vi "compressor.vi"() -> ()   [LabVIEW 2017]
uses:
  <vilib>/Rock Robotics/WPI/Utilities/WPI_GetSetVariantRefNum.vi
panel:
  out "Compressor Enabled":bool
  out "Compressor Running":bool
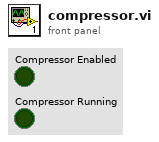
[diagram p1: front panel]
types:
  T1 = typedef "WPI_CompressorDevRef.ctl" = cluster{"DevStatus":errorcluster, "Pneumatics Control Module":u8}
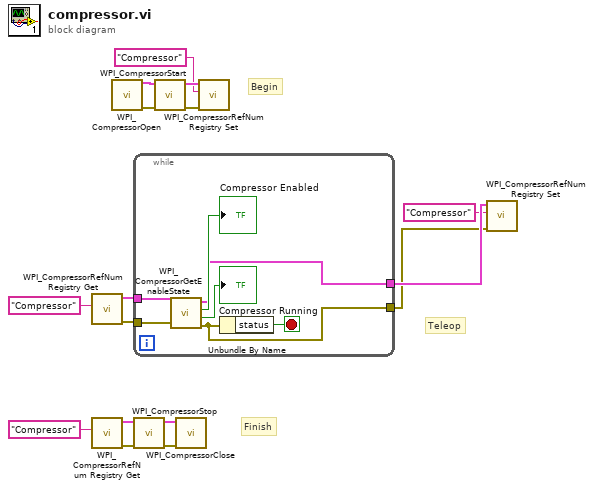
[diagram p0: block diagram]
diagram:
  # "Begin"
  # "Finish"
  # "Teleop"
  n1 = call <vilib>:"WPI_CompressorRefNum Registry Get.vi"("refnum name"="Compressor") -> ("error out"=w10:errorcluster, "CompressorDevRef"=w11:T1)  [unwired: 9 in]
  n2 = call <vilib>:"WPI_CompressorRefNum Registry Get.vi"("refnum name"="Compressor") -> ("error out"=w14:errorcluster, "CompressorDevRef"=w15:T1)  [unwired: 9 in]
  n3 = call <vilib>:"WPI_CompressorOpen.vi"() -> ("CompressorDevRef"=w7:T1, "error out"=w6:errorcluster)  [unwired: 14 in]
  n4 = while {
    tunnel: [w20] -> w9
    tunnel: w11 -> [w19]
    tunnel: w10 -> [w18]
    tunnel: [w17] -> w8
    stop <- w21 stop-if-true
    n5 = call <vilib>:"WPI_CompressorGetEnableState.vi"("error in (no error)"=w18, "CompressorDevRef"=w19) -> ("error out"=w17:errorcluster, "Compressor Running"=→"Compressor Running":bool, "Enabled"=→"Compressor Enabled":bool, "CompressorDevRef"=w20:T1)  [unwired: 6 in]
    n6 = Unbundle By Name(w17) -> ("status"=w21:bool)
  }
  n7 = call <vilib>:"WPI_CompressorStop.vi"("error in (no error)"=w14, "CompressorDevRef"=w15) -> ("error out"=w12:errorcluster, "CompressorDevRef"=w13:T1)  [unwired: 8 in]
  n8 = call <vilib>:"WPI_CompressorStart.vi"("error in (no error)"=w6, "CompressorDevRef"=w7) -> ("error out"=w4:errorcluster, "CompressorDevRef"=w5:T1)  [unwired: 8 in]
  n9 = call <vilib>:"WPI_CompressorClose.vi"("error in (no error)"=w12, "CompressorDevRef"=w13) -> ()  [unwired: 9 in, 1 out]
  n10 = call <vilib>:"WPI_CompressorRefNum Registry Set.vi"("error in (no error)"=w4, "refnum name"="Compressor", "CompressorDevRef"=w5) -> ()  [unwired: 7 in, 2 out]
  n11 = call <vilib>:"WPI_CompressorRefNum Registry Set.vi"("error in (no error)"=w8, "refnum name"="Compressor", "CompressorDevRef"=w9) -> ()  [unwired: 7 in, 2 out]
